vi "Change Description.vi"(8 "error in (no error)":errorcluster, 9 "Copy VI Descr W":bool, 10 "Description":string, 11 "VI Description W":refnum<vi>) -> (0 "error out":errorcluster)   [LabVIEW 2020]
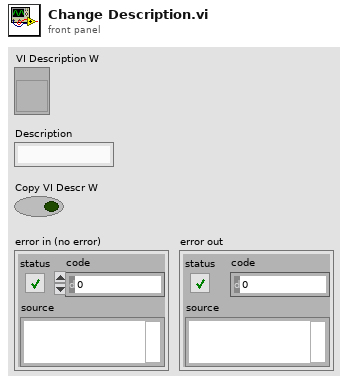
[diagram p1: front panel]
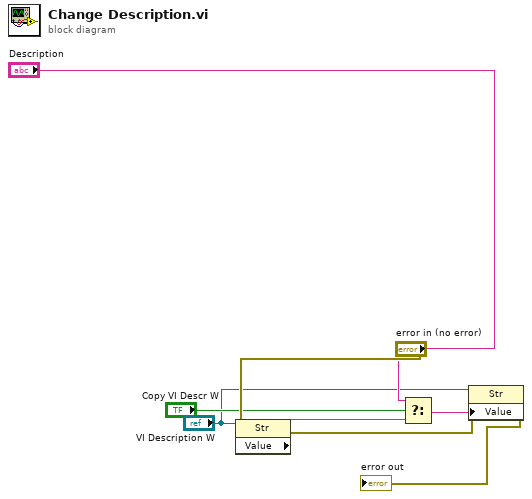
[diagram p0: block diagram]
diagram:
  n1 = property on="Property Node" class="Str"(reference="VI Description W", error in="error in (no error)") -> (error out=w7:errorcluster, "Value"=w4:string)  [unwired: 1 out]
  n2 = Select(t="Description", s="Copy VI Descr W", f=w4) -> (s? t:f=w5:string)
  n3 = property on="Property Node" class="Str"(reference="VI Description W", error in=w7, "Value"=w5) -> (error out=→"error out":errorcluster)  [unwired: 1 out]
